vi "PH_SHS_Analysis.allocate or free img space.vi"(0 "i ref in":refnum<vi>, 2 "Allocate?":bool, 5 "error in (no error)":errorcluster) -> (14 "i ref out":refnum<vi>, 19 "error out":errorcluster)   [LabVIEW 2014, in "PH_SHS_Analysis.lvlib"]
doc: "This VI is forseen to be used in constructor or destructor. If Allocate? = true is chosen, memory space for several images is allocated. If false is chosen, it is freed."
uses:
  PH_SHS_Analysis.lvlib
  CS_Core/CSSystem/CSSystemLib/CSSystemLib.lvlib
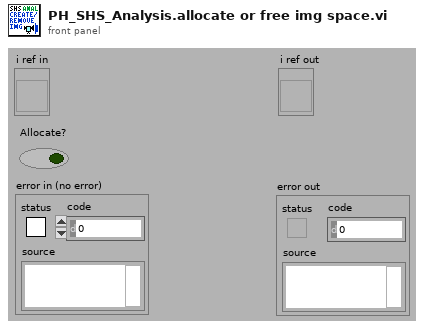
[diagram p1: front panel]
types:
  T1 = typedef "PH_SHS_Analysis.lvlib/PH_SHS_Analysis.i attribute.ctl" = cluster{"GUI Refs":cluster{"Delete":refnum<vi>, "Global On":refnum<vi>, "Cam Source":refnum<vi>, "Calibration Data File":refnum<vi>, "Calibration status":refnum<vi>, "Show overlay":refnum<vi>, "SHS Device Config":refnum<vi>, "Result":refnum<vi>, "Consider Tilt":refnum<vi>, "Working Reference":refnum<vi>, "Remove Tilt":refnum<vi>, "Take Cali  Reference":refnum<vi>, "Publishing Data Status":refnum<vi>, "Calibration Data":refnum<vi>}, "Calibration":cluster{"Status":T2, "Data":T3, "File":path}, "Result":T8, "Image":T11, "SHS Device Config":T12, "Show Overlay":bool, "GradientZernikeMatrix":dbl[][], "Consider Tilt":bool, "Working Reference":T4, "Zernicke Service ID":i32, "PSDB Image":T11}
  T2 = typedef "PH_StatusHandler.lvlib/PH_StatusHandler.Status.ctl" = i16
  T3 = typedef "PH_SHS_Analysis_Calibrator.lvlib/PH_SHS_Analysis_Calibrator.Analysis Calibration Data.ctl" = cluster{"Date":string, "Time":string, "Cam Settings":cluster{"Cam ID":string, "Gain":dbl, "Brightness":dbl, "Shutter":dbl, "Cam Error":bool, "Mode":i32}, "SHS Reference Result":T4, "Pixel Size":dbl, "MLA Pitch":dbl, "Method":enum16{"automatic", "manual"}, "Calibration Data calculated":bool, "No Problems at calculation?":bool, "error out":errorcluster}
  T4 = typedef "SHS_Common.lvlib/SHSReference.ctl" = cluster{"Reference":T5[][], "Lens Array Pitch [px]":dbl}
  T5 = typedef "SHS_Common.lvlib/ReferencePoint.ctl" = cluster{"Rect":T6, "Point":T7}
  T6 = typedef "SHS_Common.lvlib/Rectangle.ctl" = cluster{"Left":i32, "Top":i32, "Right":i32, "Bottom":i32}
  T7 = typedef "SHS_Common.lvlib/Point.ctl" = cluster{"x":dbl, "y":dbl, "valid?":bool, "weight":dbl}
  T8 = typedef "PH_SHS_Analysis.lvlib/PH_SHS_Analysis.Result.ctl" = cluster{"Time Stamp":timestamp, "Zernike Coefficients":T9, "PtV [lambda]":dbl, "Shifts":T10, "Measurement Quality":cluster{dbl, dbl, dbl}, "Measurement valid?":bool}
  T9 = typedef "PH_SHS_Analysis.lvlib/PH_SHS_Analysis.Zernike Coefficients.ctl" = cluster{"Tilt x":dbl, "Tilt y":dbl, "Defocus":dbl, "Astig 0°":dbl, "Astig 45°":dbl, "Coma x":dbl, "Coma y":dbl, "Spherical":dbl, "Trefoil 0°":dbl, "Trefoil 30°":dbl, "2nd Astig 0°":dbl, "2nd Astig 45°":dbl, "2nd Coma x":dbl, "2nd Coma y":dbl, "2nd Spherical":dbl}
  T10 = typedef "SHS_Common.lvlib/Shifts.ctl" = T7[][]
  T11 = typedef "IMAQ Image.ctl" = refnum<image>
  T12 = typedef "SHS_Analysis.lvlib/SHS_DeviceConfig.ctl" = cluster{"focal length [m]":dbl, "pixel size [m/px]":dbl, "wavelength [m]":dbl}
  T13 = typedef "Image Type" = u32
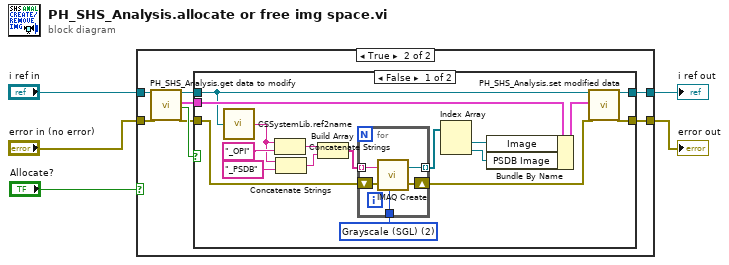
[diagram p0: block diagram]
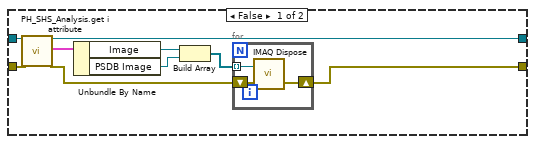
[diagram p2: hidden frame]
diagram:
  n1 = case shown="True" "Allocate?" {
    tunnel: [w9 w24] -> w5
    tunnel: [w11 w23] -> w4
    tunnel: "error in (no error)" -> [w14 w20]
    tunnel: "i ref in" -> [w13 w19]
    frame False {
      n2 = call "PH_SHS_Analysis.get i attribute.vi"("i ref in"=w13, "error in (no error)"=w14) -> ("i ref out"=w11:refnum<vi>, "i attribute"=w12:T1, "error out"=w10:errorcluster)  [unwired: 15 in]
      n3 = Unbundle By Name(w12) -> ("Image"=w8:T11, "PSDB Image"=w6:T11)
      n4 = Build Array(w8, w6) -> (w7:T11[])
      n5 = for {
        tunnel: w7 -> [w15] mode=indexing
        shift-right: [w16] -> w9
        shift-left: w10 -> [w17]
        n6 = call "IMAQ Dispose"("Image"=w15, "error in (no error)"=w17) -> ("error out"=w16:errorcluster)  [unwired: 4 in]
      }
    }
    frame True {
      n7 = call "PH_SHS_Analysis.get data to modify.vi"("i ref in"=w19, "error in (no error)"=w20) -> ("i ref out"=w22:refnum<vi>, "i attribute"=w18:T1, "timed out"=w25:bool, "error out"=w21:errorcluster)  [unwired: 14 in]
      n8 = case shown="False" w25 {
        tunnel: w21 -> [w37 w48]
        tunnel: w22 -> [w35 w49]
        tunnel: [w42 w49] -> w23
        tunnel: [w41 w48] -> w24
        tunnel: w18 -> [w40 _]
        frame False {
          w36 = T13 2 items=["Grayscale (U8)", "Grayscale (I16)", "Grayscale (SGL)", "Complex (CSG)", "RGB (U32)", "HSL (U32)", "RGB (U64)"] ("Image Type")
          n9 = call "CSSystemLib.ref2name.vi"("obj refnum"=w35) -> ("name"=w32:string)
          n10 = Concatenate Strings(w32, "_OPI") -> (w34:string)
          n11 = Concatenate Strings(w32, "_PSDB" ("string")) -> (w29:string)
          n12 = Build Array(w34, w29) -> (w30:string[])
          n13 = for {
            tunnel: w36 -> [w45]
            tunnel: w30 -> [w44] mode=indexing
            tunnel: [w43] -> w28 mode=indexing
            shift-right: [w47] -> w38
            shift-left: w37 -> [w46]
            n14 = call "IMAQ Create"("Image Name"=w44, "Image Type"=w45, "error in (no error)"=w46) -> ("New Image"=w43:T11, "error out"=w47:errorcluster)  [unwired: 2 in]
          }
          n15 = Index Array(array=w28) -> (element #1=w27:T11, element #2=w26:T11)  [unwired: 2 in]
          n16 = Bundle By Name(cluster=w40, "Image"=w27, "PSDB Image"=w26) -> (w39:T1)
          n17 = call "PH_SHS_Analysis.set modified data.vi"("i ref in"=w35, "i attribute"=w39, "error in (no error)"=w38) -> ("i ref out"=w42:refnum<vi>, "error out"=w41:errorcluster)  [unwired: 15 in]
        }
        frame True {
        }
      }
    }
  }
  "error out" <- w5
  "i ref out" <- w4
